vi "Check Host Creds Exist.vi"(8 "error in (no error)":errorcluster, 10 "Host":string) -> (0 "error out":errorcluster, 2 "Exists":bool)   [LabVIEW 2020, in "GPack.lvlib" / "GPackPrefs.lvclass"]
uses:
  GPackPrefs.lvclass
  <vilib>/Utility/config.llb/Read Key (String).vi
  GPackPrefs.lvclass/GPackPrefs.ctl
  <vilib>/Utility/config.llb/NI_LVConfig.lvlib
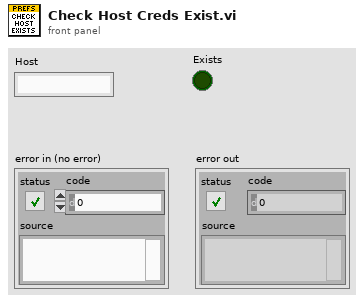
[diagram p1: front panel]
types:
  T1 = typedef "NI_LVConfig.lvlib/Config Data RefNum.ctl" = refnum<k1>
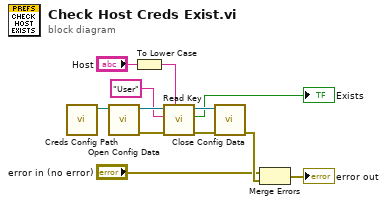
[diagram p0: block diagram]
diagram:
  n1 = call "Creds Config Path.vi"() -> ("Creds Config Path"=w12:path)  [unwired: 11 in]
  n2 = call <vilib>:"Open Config Data.vi"("configuration file path"=w12) -> ("error out"=w7:errorcluster, "refnum"=w11:T1)  [unwired: 8 in, 1 out]
  n3 = To Lower Case(string="Host") -> (all lower case string=w8:string)
  n4 = call-poly <vilib>:"Read Key.vi"("section"=w8, "error in (no error)"=w7, "key"="User", "refnum"=w11) -> ("error out"=w5:errorcluster, "found?"=→"Exists":bool, "refnum out"=w6:T1)  [unwired: 4 in, 1 out]
  n5 = call <vilib>:"Close Config Data.vi"("error in (no error)"=w5, "refnum"=w6) -> ("error out"=w3:errorcluster)  [unwired: 8 in, 1 out]
  n6 = Merge Errors("error in (no error)", w3) -> (→"error out":errorcluster)
